vi "LJM logger open with invalid device type filter.vi"(4 "error in":errorcluster, 5 "DeviceType":string="LJM_dtANY", 6 "ConnectionType":string="LJM_ctANY", 7 "Identifier":string) -> (0 "error out":errorcluster, 3 "Handle":i32)   [LabVIEW 2026]
panel:
  # "The loggers allow a few invalid names for the device type string reported to the user, so this VI  filters/reshapes those bad names to valid parameters."
  # "Be sure to change LJM logger open constants to string.vi and LJM logger get error open params.vi if you change this VI."
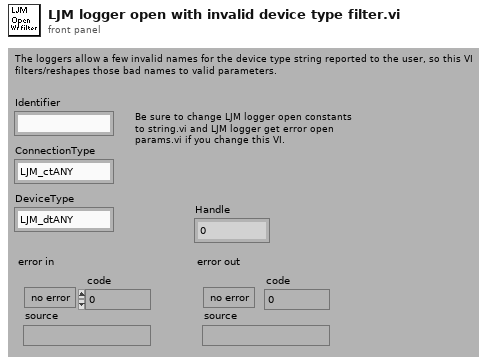
[diagram p1: front panel]
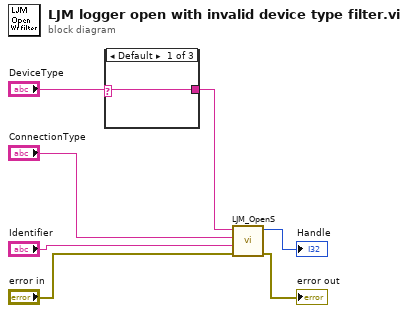
[diagram p0: block diagram]
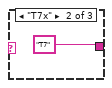
[diagram p2: hidden frame]
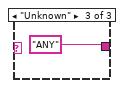
[diagram p3: hidden frame]
diagram:
  n1 = case shown="Default" "DeviceType" {
    selector: "DeviceType" -> [w8 _ _]
    tunnel: [w8 "T7" "ANY"] -> w4
    frame Default {
    }
    frame "T7x" {
    }
    frame "Unknown" {
    }
  }
  n2 = call "LJM_OpenS.vi"("error in"="error in", "Identifier"="Identifier", "ConnectionType"="ConnectionType", "DeviceType"=w4) -> ("error out"=→"error out":errorcluster, "Handle"=→"Handle":i32)  [unwired: 6 in]
